vi "Valid Range or Not.vi"(8 "error in (no error)":errorcluster, 9 "end position":cluster{"row":i8, "column":i8}, 10 "start position":cluster{"row":i8, "column":i8}, 11 "cluster of private data in":T1={"FPGA VI Reference"=refnum, "device index"=0, "screen size"=enum."8x1", "font size"=enum."5x8", "auto wrap"=FALSE, "alignment"=enum."None", "number of line"=enum."2 lines", "shift 0"=0, "entry mode 0"=enum."increment & no shift", "shift 1"=0, "entry mode 1"=enum."increment & no shift"}) -> (0 "error out":errorcluster, 1 "end position out":cluster{"row":i8, "column":i8}, 2 "start position out":cluster{"row":i8, "column":i8}, 3 "cluster of private data out":T1={"FPGA VI Reference"=refnum, "device index"=0, "screen size"=enum."8x1", "font size"=enum."5x8", "auto wrap"=FALSE, "alignment"=enum."None", "number of line"=enum."2 lines", "shift 0"=0, "entry mode 0"=enum."increment & no shift", "shift 1"=0, "entry mode 1"=enum."increment & no shift"})   [LabVIEW 2017, in "HD44780.lvclass"]
uses:
  HD44780.lvclass
  Common/HD44780 Common.lvlib
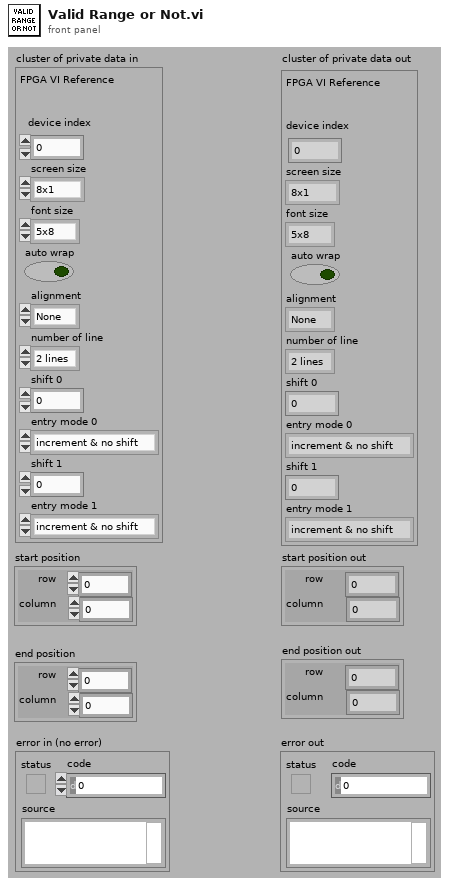
[diagram p1: front panel]
types:
  T1 = cluster{"FPGA VI Reference":refnum<k20>, "device index":i8, "screen size":enum8{"8x1", "8x2", "12x4", "16x1", "16x2", "16x4", "20x1", "20x2", "20x4", "24x1", "24x2", "40x2", "40x4"}, "font size":enum8{"5x8", "5x10"}, "auto wrap":bool, "alignment":enum16{"None", "Left", "Center", "Right"}, "number of line":enum8{"1 line", "2 lines"}, "shift 0":i8, "entry mode 0":enum8{"increment & no shift", "increment & shift", "decrement & no shift", "decrement & shift"}, "shift 1":i8, "entry mode 1":enum8{"increment & no shift", "increment & shift", "decrement & no shift", "decrement & shift"}}
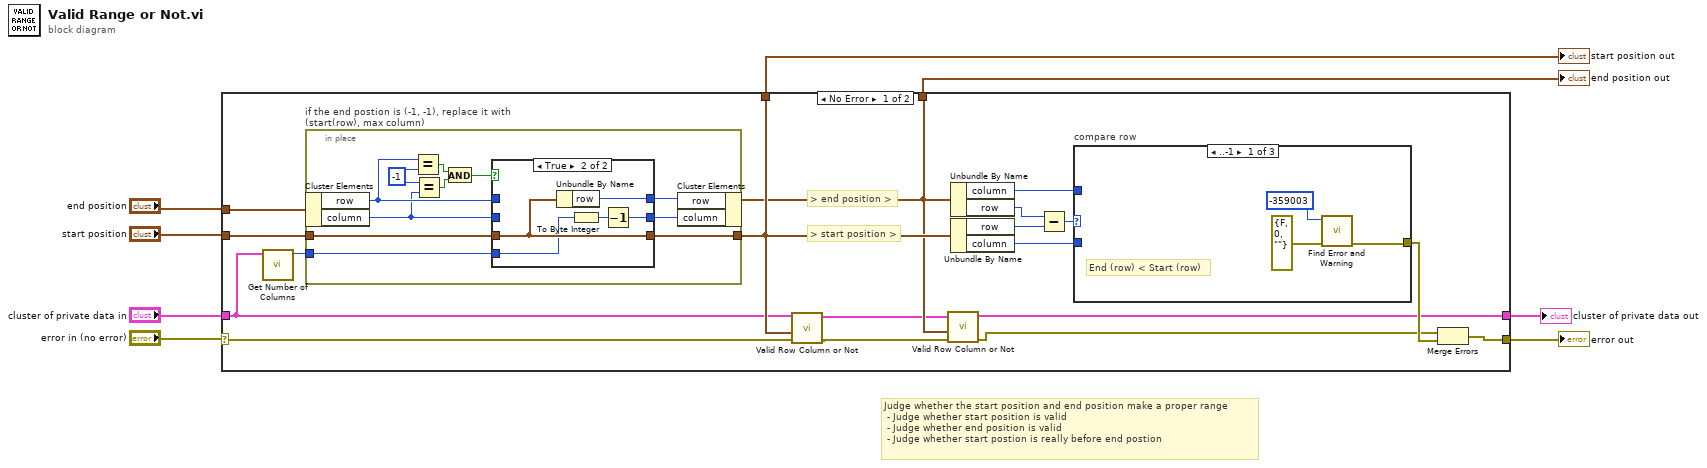
[diagram p0: block diagram]
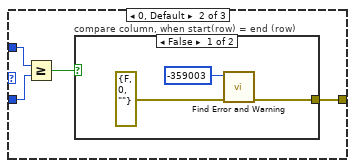
[diagram p2: hidden frame]
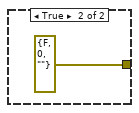
[diagram p3: hidden frame]
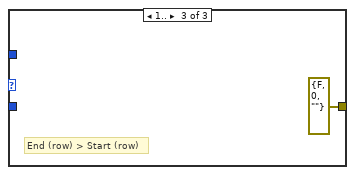
[diagram p4: hidden frame]
diagram:
  # "Judge whether the start position and end position make a proper range\n - Judge whether start position is valid\n - Judge whether end position is valid\n - Judge whether start postion is really before end postion"
  n1 = case shown="No Error" "error in (no error)" {
    selector: "error in (no error)" -> [w26 w59]
    tunnel: [w25 w59] -> w7
    tunnel: "end position" -> [w24 w60]
    tunnel: "start position" -> [w16 w61]
    tunnel: [w14 w60] -> w4
    tunnel: [w15 w61] -> w3
    tunnel: "cluster of private data in" -> [w9 w58]
    tunnel: [w12 w58] -> w1
    frame No Error {
      # "> start position >"
      # "> end position >"
      n2 = call "Get Number of Columns.vi"("cluster of private data in"=w9) -> ("column number"=w23:u8)  [unwired: 10 in]
      n3 = in-place "if the end postion is (-1, -1), replace it with (start(row), max column)" {
        in-place-border: w16 -> [w41]
        in-place-border: [w40] -> w15
        in-place-border: w23 -> [w39]
        w49 = i8 -1 ("y")
        n4 = in-place-cluster #1(w24) -> ("row"=w44:i8, "column"=w42:i8)
        n5 = Equal?(x=w44, y=w49) -> (x = y?=w48:bool)
        n6 = Equal?(x=w49, y=w42) -> (x = y?=w47:bool)
        n7 = And(x=w48, y=w47) -> (x .and. y?=w46:bool)
        n8 = case shown="True" w46 {
          tunnel: [w52 w57] -> w45
          tunnel: w44 -> [w52 _]
          tunnel: [w51 w53] -> w43
          tunnel: w42 -> [w51 _]
          tunnel: w41 -> [w50 w56]
          tunnel: [w50 w56] -> w40
          tunnel: w39 -> [_ w54]
          frame False {
          }
          frame True {
            n9 = Unbundle By Name(w56) -> ("row"=w57:i8)
            n10 = To Byte Integer(number=w54) -> (8bit integer=w55:i8)
            n11 = Decrement(x=w55) -> (x-1=w53:i8)
          }
        }
        n12 = in-place-cluster #1("row"=w45, "column"=w43) -> (w14:cluster{"row":i8, "column":i8})
      }
      n13 = call "Valid Row Column or Not.vi"("error in (no error)"=w26, "cursor position in"=w15, "cluster of private data in"=w9) -> ("error out"=w11:errorcluster, "cluster of private data out"=w13:T1)  [unwired: 6 in, 1 out]
      n14 = call "Valid Row Column or Not.vi"("error in (no error)"=w11, "cursor position in"=w14, "cluster of private data in"=w13) -> ("error out"=w10:errorcluster, "cluster of private data out"=w12:T1)  [unwired: 6 in, 1 out]
      n15 = Unbundle By Name(w14) -> ("column"=w18:i8, "row"=w17:i8)
      n16 = Unbundle By Name(w15) -> ("row"=w20:i8, "column"=w22:i8)
      n17 = Subtract(x=w17, y=w20) -> (x-y=w19:i8)
      n18 = case "compare row" shown="..-1" w19 {
        tunnel: w18 -> [_ w33 _]
        tunnel: w22 -> [_ w32 _]
        tunnel: [w27 w30 errorcluster {"status"=FALSE, "code"=0, "source"=""} ("error in")] -> w21
        frame ..-1 {
          # "End (row) < Start (row)"
          n19 = call "Find Error and Warning.vi"("error in (no error)"=errorcluster {"status"=FALSE, "code"=0, "source"=""}, "error code"=-359003) -> ("error out"=w27:errorcluster)  [unwired: 9 in]
        }
        frame 0, Default {
          n20 = Greater Or Equal?(x=w33, y=w32) -> (x >= y?=w31:bool)
          n21 = case "compare column, when start(row) = end (row)" shown="False" w31 {
            tunnel: [w36 errorcluster {"status"=FALSE, "code"=0, "source"=""} ("error in")] -> w30
            frame False {
              n22 = call "Find Error and Warning.vi"("error in (no error)"=errorcluster {"status"=FALSE, "code"=0, "source"=""}, "error code"=-359003) -> ("error out"=w36:errorcluster)  [unwired: 9 in]
            }
            frame True {
            }
          }
        }
        frame 1.. {
          # "End (row) > Start (row)"
        }
      }
      n23 = Merge Errors(w10, w21) -> (w25:errorcluster)
    }
    frame Error {
    }
  }
  "cluster of private data out" <- w1
  "error out" <- w7
  "start position out" <- w3
  "end position out" <- w4
